vi "Meas and Calculation.vi"(5 "Beam Size Percentage":dbl=5.0, 7 "Beam Size Target":dbl=3.125, 8 "error in (no error)":errorcluster, 9 "Circularity_min":dbl=95.0, 10 "Peak Resp_min":dbl=95.0, 11 "Beam Profiler in":refnum<class "Beam Profiler.lvclass">) -> (0 "error out":errorcluster caption="error out (no error)", 1 "BV Data":T1={"Centroid X[um]"=nan, "Centroid Y[um]"=nan, "PeakResp.[%]"=nan, "Knife Edge X[mm]"=nan, "Knife Edge Y[mm]"=nan, "Circularity"=nan, "Collimation Result"=FALSE} {"PeakResp.[%]" format="%.0g"}, 2 "Collimation result":bool, 3 "Beam Profiler out":refnum<class "Beam Profiler.lvclass">)   [LabVIEW 2018]
uses:
  State data/BV Data.ctl
  <instrlib>/nLight Instruments/Beam Profiler/Beam Profiler.lvclass
  State data/Fiber Auto Collimation state data.lvclass
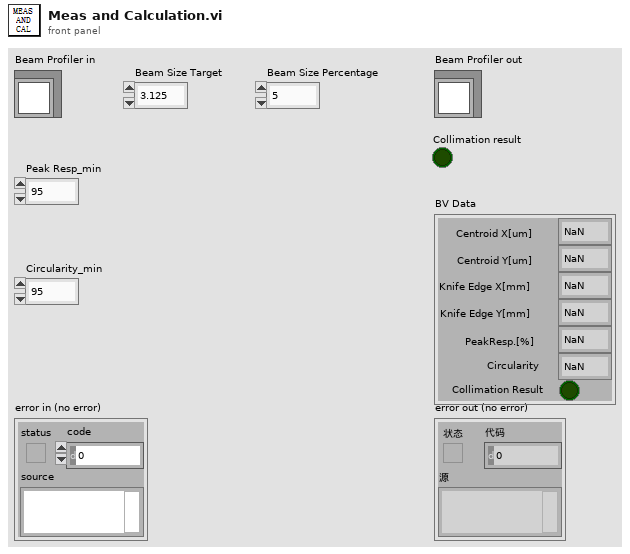
[diagram p1: front panel]
types:
  T1 = typedef "Fiber Auto Collimation state data.lvclass/BV Data.ctl" = cluster{"Centroid X[um]":sgl, "Centroid Y[um]":sgl, "PeakResp.[%]":dbl, "Knife Edge X[mm]":sgl, "Knife Edge Y[mm]":sgl, "Circularity":sgl, "Collimation Result":bool}
  T2 = typedef "Beam Profiler.lvclass/Beam profiler XY distance value pair.ctl" = cluster{"X":dbl[unit], "Y":dbl[unit]}
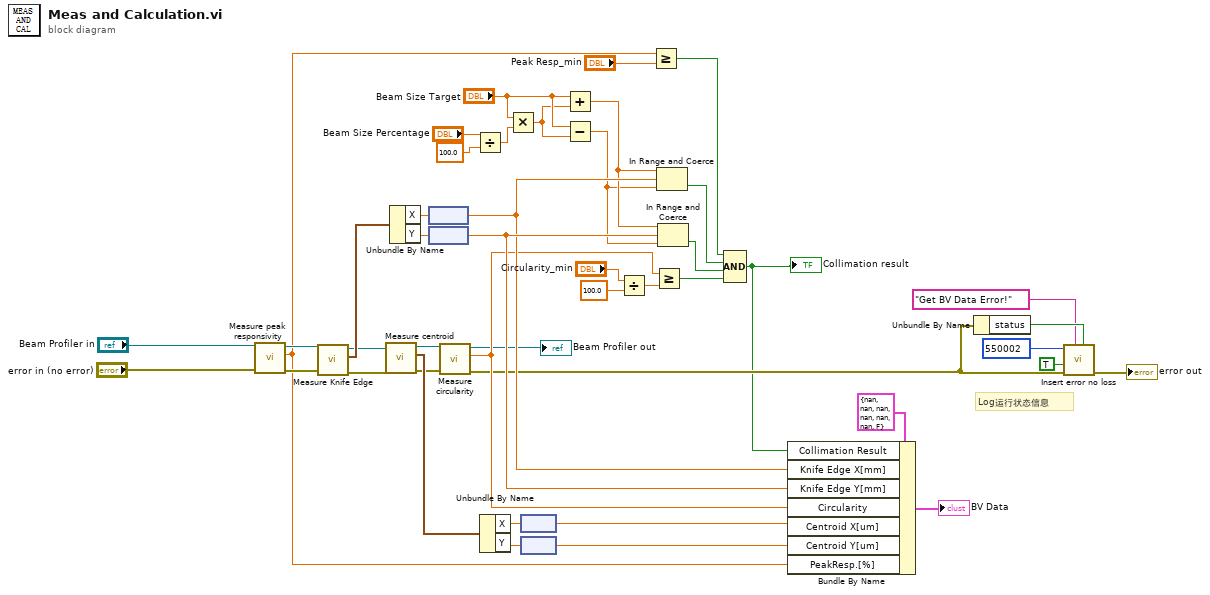
[diagram p0: block diagram]
diagram:
  # "Log运行状态信息"
  n1 = call-dynamic "Measure peak responsivity.vi"("error in (no error)"="error in (no error)", "Beam Profiler in"="Beam Profiler in") -> ("error out"=w45:errorcluster, "Peak responsivity [%,0-100]"=w30:dbl, "Beam Profiler out"=w44:refnum<class "Beam Profiler.lvclass">)  [unwired: 7 in]
  n2 = call-dynamic "Measure Knife Edge.vi"("error in (no error)"=w45, "Beam Profiler 输入"=w44) -> ("error out"=w39:errorcluster, "Knife Edge"=w43:T2, "Beam Profiler 输出"=w40:refnum<class "Beam Profiler.lvclass">)  [unwired: 7 in]
  n3 = call-dynamic "Measure centroid.vi"("error in (no error)"=w39, "Beam Profiler in"=w40) -> ("error out"=w25:errorcluster, "Centroid location"=w35:T2, "Beam Profiler out"=w24:refnum<class "Beam Profiler.lvclass">)  [unwired: 7 in]
  n4 = Unbundle By Name(w43) -> ("X"=w32:dbl[unit], "Y"=w31:dbl[unit])
  n5 = node(w32) -> (w26:dbl)
  n6 = node(w31) -> (w27:dbl)
  n7 = call-dynamic "Measure circularity.vi"("error in (no error)"=w25, "Beam Profiler 输入"=w24) -> ("error out"=w5:errorcluster, "Circularity"=w22:dbl, "Beam Profiler 输出"=→"Beam Profiler out":refnum<class "Beam Profiler.lvclass">)  [unwired: 7 in]
  n8 = Divide(x="Beam Size Percentage", y=100.0) -> (x/y=w19:dbl)
  n9 = Unbundle By Name(w35) -> ("X"=w34:dbl[unit], "Y"=w33:dbl[unit])
  n10 = Multiply(x="Beam Size Target", y=w19) -> (x*y=w17:dbl)
  n11 = node(w34) -> (w29:dbl)
  n12 = node(w33) -> (w28:dbl)
  n13 = Add(x="Beam Size Target", y=w17) -> (x+y=w16:dbl)
  n14 = Subtract(x="Beam Size Target", y=w17) -> (x-y=w15:dbl)
  n15 = Divide(x="Circularity_min", y=100.0) -> (x/y=w11:dbl)
  n16 = Greater Or Equal?(x=w30, y="Peak Resp_min") -> (x >= y?=w38:bool)
  n17 = Greater Or Equal?(x=w22, y=w11) -> (x >= y?=w21:bool)
  n18 = In Range and Coerce(upper limit=w16, x=w26, lower limit=w15) -> (In Range?=w42:bool)  [unwired: 1 out]
  n19 = In Range and Coerce(upper limit=w16, x=w27, lower limit=w15) -> (In Range?=w41:bool)  [unwired: 1 out]
  n20 = Compound Arithmetic op=AND ("复合运算")(w38, w42, w41, w21) -> (w4:bool)
  "Collimation result" <- w4
  n21 = Bundle By Name(cluster=T1 {"Centroid X[um]"=nan, "Centroid Y[um]"=nan, "PeakResp.[%]"=nan, "Knife Edge X[mm]"=nan, "Knife Edge Y[mm]"=nan, "Circularity"=nan, "Collimation Result"=FALSE} ("BV Data"), "Collimation Result"=w4, "Knife Edge X[mm]"=w26, "Knife Edge Y[mm]"=w27, "Circularity"=w22, "Centroid X[um]"=w29, "Centroid Y[um]"=w28, "PeakResp.[%]"=w30) -> (→"BV Data":T1)
  n22 = Unbundle By Name(w5) -> ("status"=w9:bool)
  n23 = call <userlib>:"Insert error no loss.vi"("Add error? (T)"=w9, "error message"="Get BV Data Error!" ("format string"), "error in (no error)"=w5, "Error = T, Warning = F (T)"=TRUE, "error code"=550002) -> ("error out"=→"error out":errorcluster)  [unwired: 4 in]
